vi "AlGaInPAs_prep_run_cont_dil_v14.vi"(2 "Debug Mode":bool, 3 "Elapsed Time(s)":dbl, 4 "State":enum16{"Edit", "Start", "Run", "End", "Idle"}(ring), 5 "Argument List In":string[](array[string])) -> (0 "Status Out":string, 1 "Argument List Out":string[](array[string]))   [LabVIEW 2011]
panel:
  out "Prep-In var":bool
  out "Prep-Ga var":bool
  out "Prep-Al var":bool
  out "Prep-P var":bool
  out "Prep-As var":bool
  out "prep_done":bool
  out "run started":bool
  out "first":bool=TRUE
  out "total time":dbl
  out "is OK?":bool
  out "AsH3?":bool
  out "PH3?":bool
  out "In?":bool
  out "Ga?":bool
  out "Al?":bool
  in  "Prep As":bool caption="Pre-run"
  in  "Prep P":bool caption="Pre-run"
  in  "Prep In":bool caption="Pre-run"
  in  "prep_time":dbl caption="pre-run time (s)"
  in  "Prep Al":bool caption="Pre-run"
  in  "Run As":bool caption="Run"
  in  "AsH3 Flow":dbl caption="AsH3 Flow (0-10 sccm)" format="%.2f"
  in  "P Flow":dbl caption="P Flow (0-100 sccm)" format="%.2f"
  in  "Run P":bool caption="Run"
  in  "In Flow":dbl caption="In Flow (0-100 sscm)" format="%.2f"
  in  "Run In":bool caption="Run"
  in  "Run Al":bool caption="Run"
  in  "Al Flow":dbl caption="Al Flow (0-100 sscm)" format="%.2f"
  in  "Cancel":bool
  in  "OK":bool
  out "tTotal(s) 2":dbl
  in  "Ga Tab Control":enum32{"Page 1", "Page 2", "Page 3"}(tab)
  in  "Ga Dilution":bool caption="Dilute"
  in  "Ga Flow set":dbl=1.0 caption="Ga Flow (0-10 sscm)" format="%.4f"
  in  "Run Ga":bool caption="Run"
  in  "Prep Ga":bool caption="Pre-run"
  out "Ga Flow val":dbl caption="Ga Flow (0-10 sscm)" format="%.2f"
  in  "GAMFC1 set":dbl=1.0 caption="R1 (0-10 sscm)" format="%.2f"
  in  "GAMFC3 set":dbl=100.0 caption="R3 (0-1000 sscm)" format="%.1f"
  out "GAMFC1 val":dbl caption="R1 (0-10 sscm)" format="%.2f"
  in  "GAMFC2 set":dbl=10.0 caption="R2 (0-100 sscm)" format="%.2f"
  out "GAMFC3 val":dbl=100.0 caption="R3 (0-1000 sscm)" format="%.1f"
  out "GAMFC2 val":dbl caption="R2 (0-100 sscm)" format="%.2f"
  in  "Ga calculated":u16(ring) items=["Ga flow", "MFC1", "MFC2", "MFC3"]
  # "Add pre-run time to run time in editor."
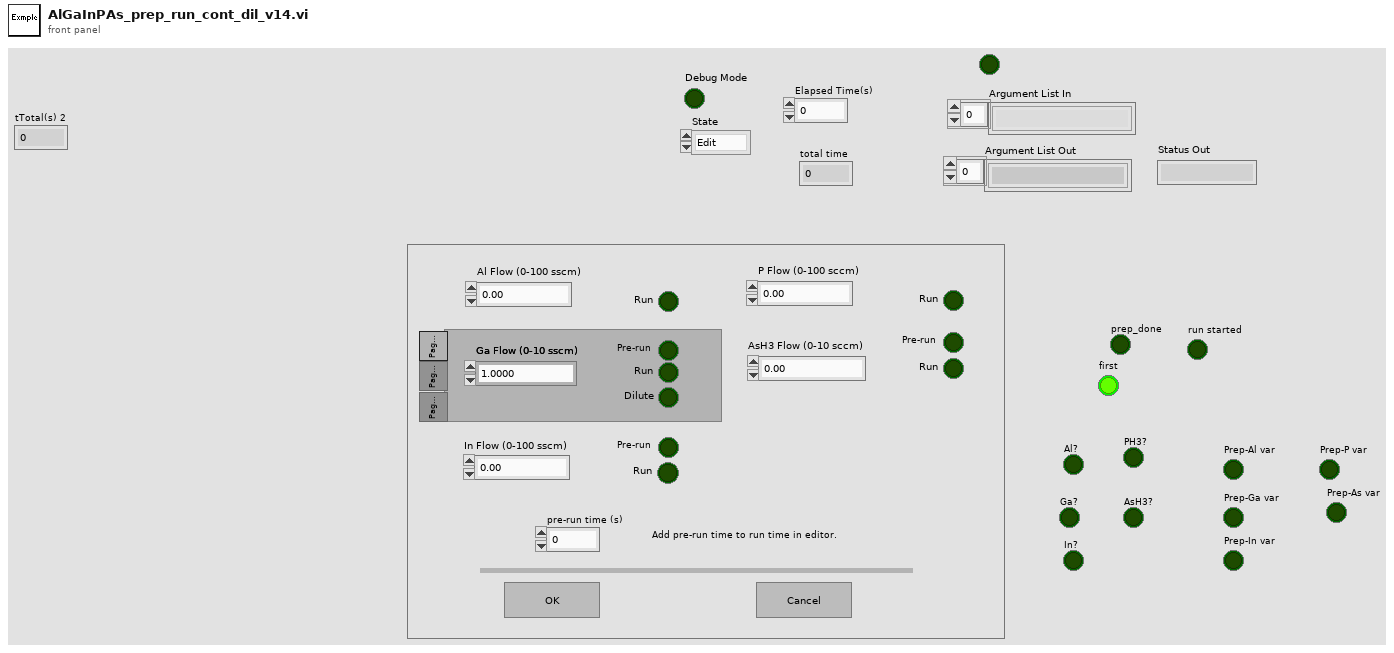
[diagram p1: front panel]
types:
  T1 = enum16{"Discrete", "Continuous", "Instantaneous", "Finite"}
  T2 = enum32{"Invalid", "Default", "Floating", "Floating/Auto-Hide", "Modal"}
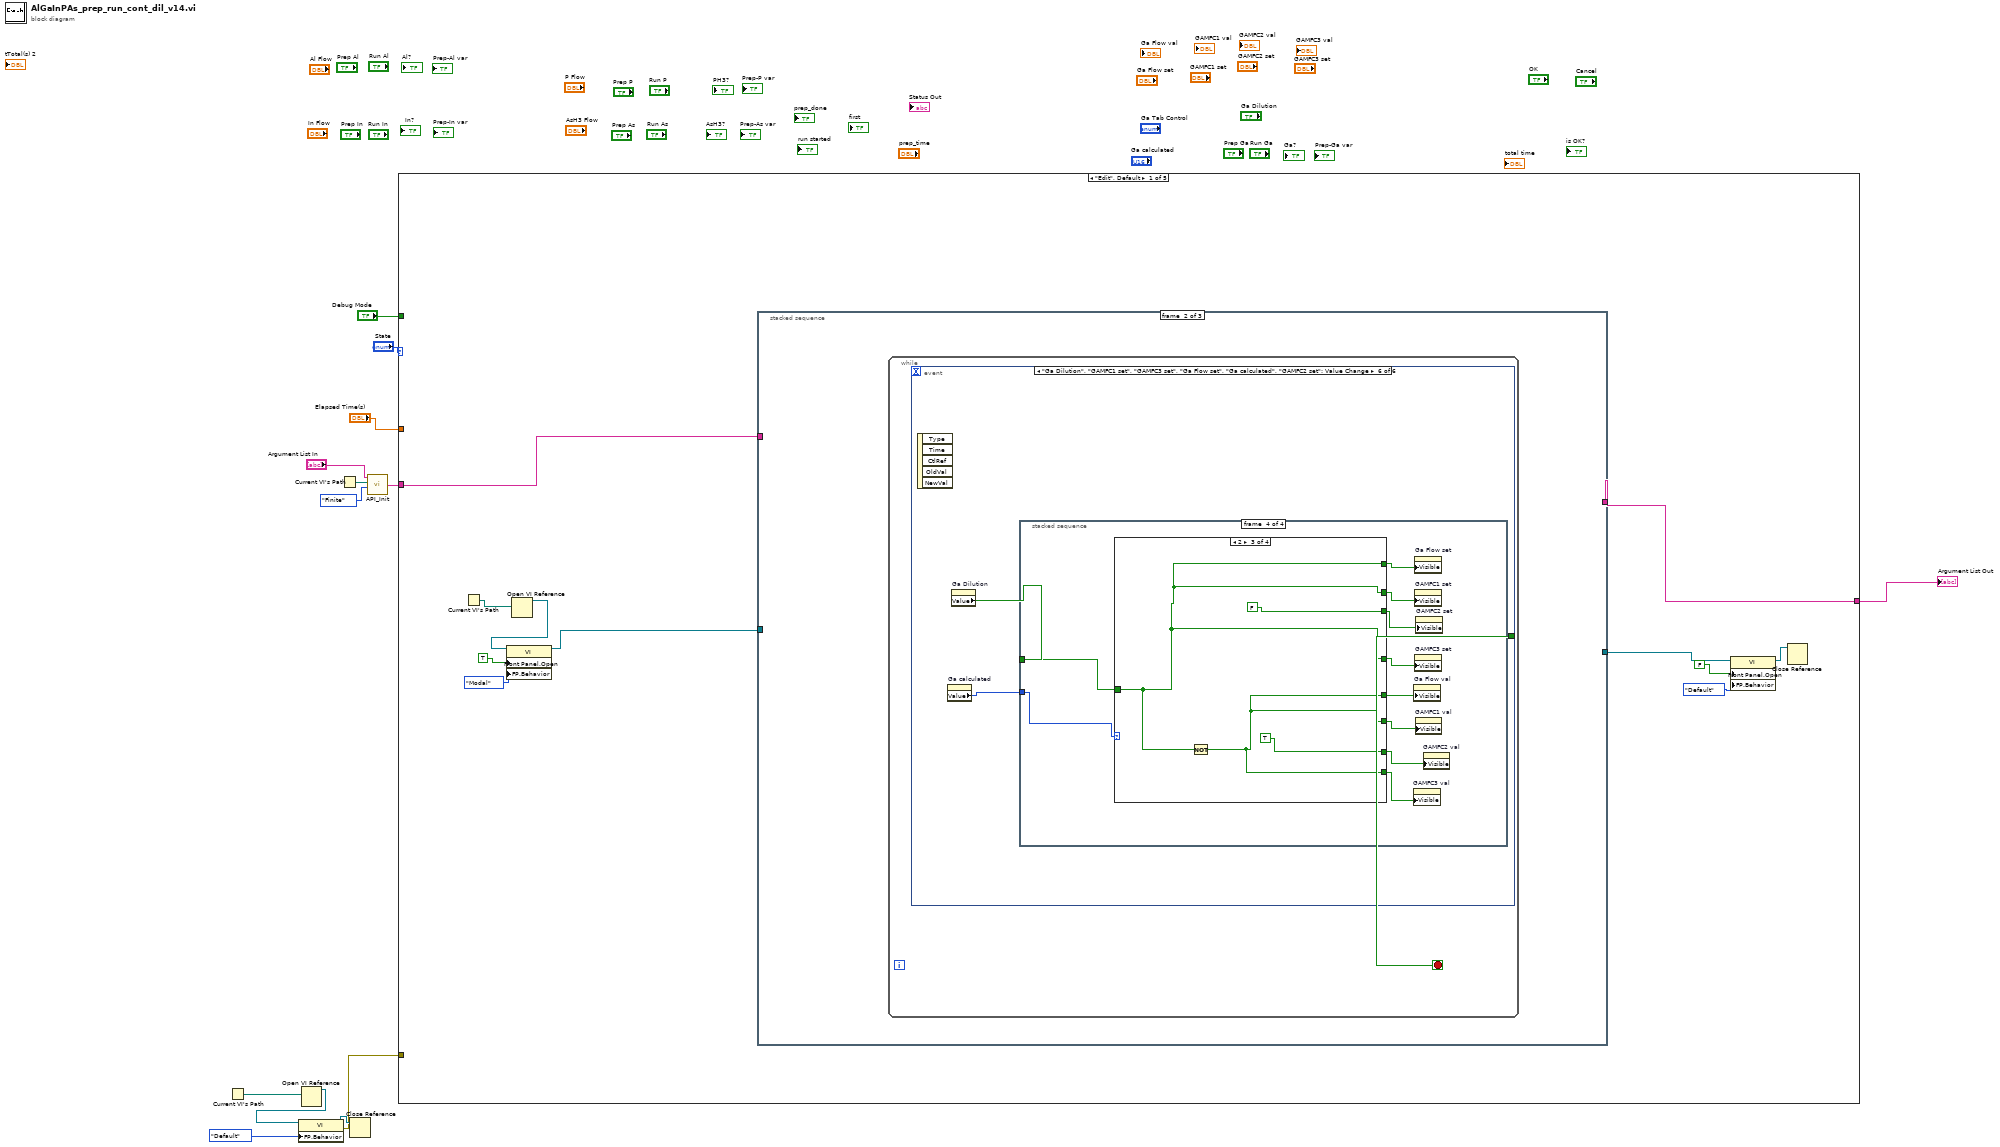
[diagram p0: block diagram]
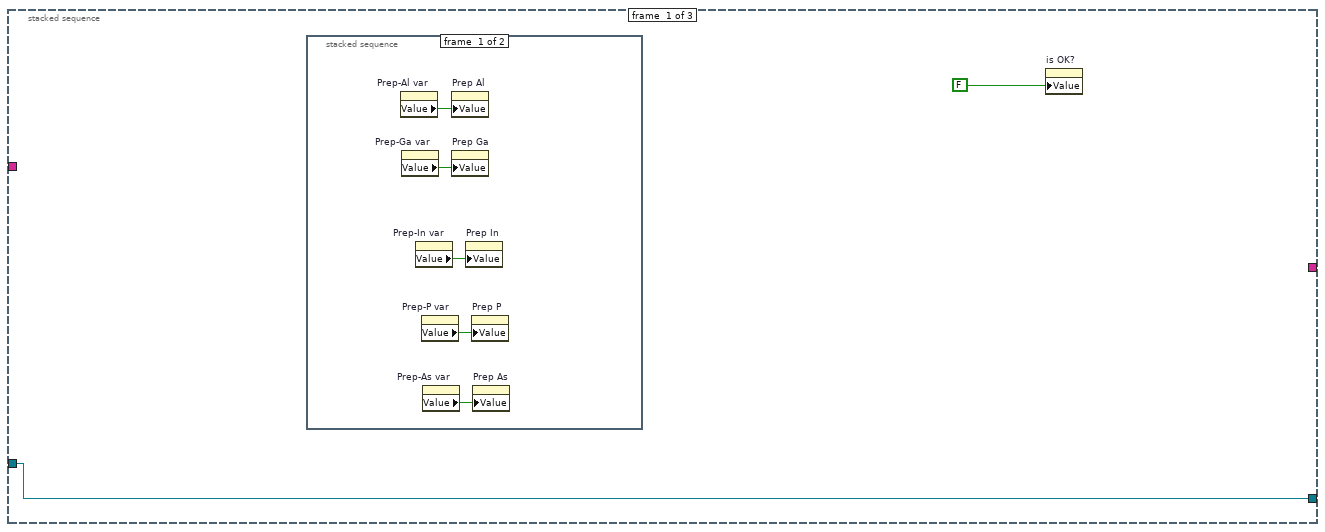
[diagram p2: hidden frame]
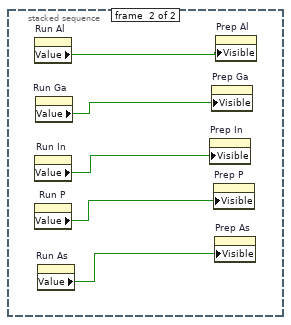
[diagram p3: hidden frame]
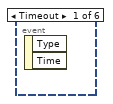
[diagram p4: hidden frame]
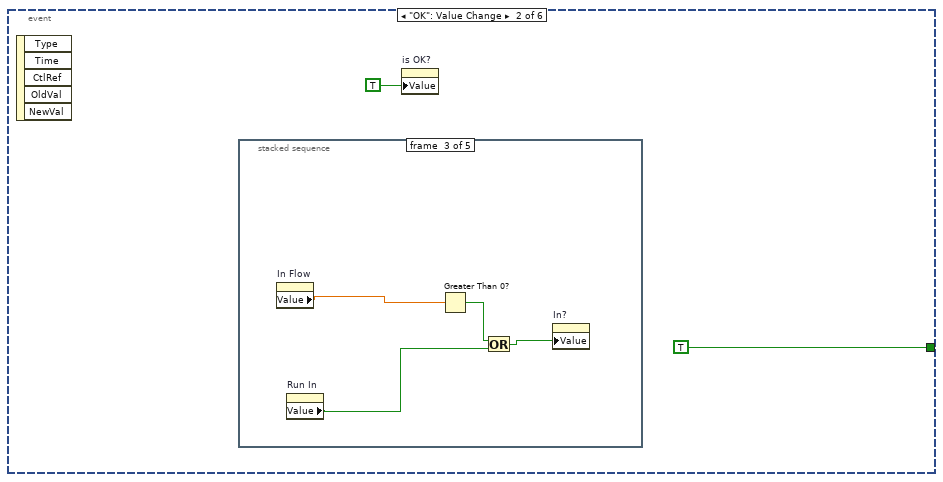
[diagram p5: hidden frame]
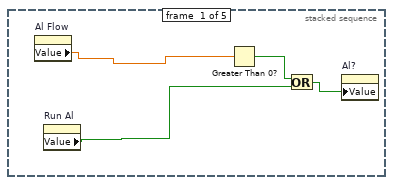
[diagram p6: hidden frame]
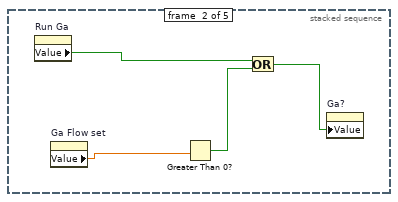
[diagram p7: hidden frame]
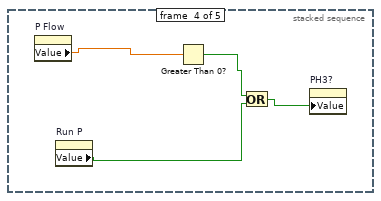
[diagram p8: hidden frame]
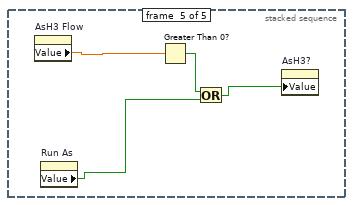
[diagram p9: hidden frame]
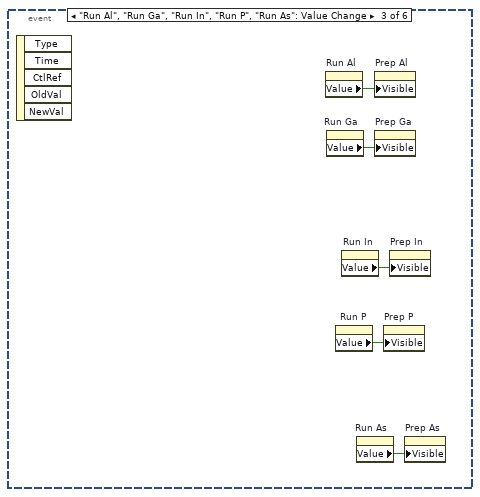
[diagram p10: hidden frame]
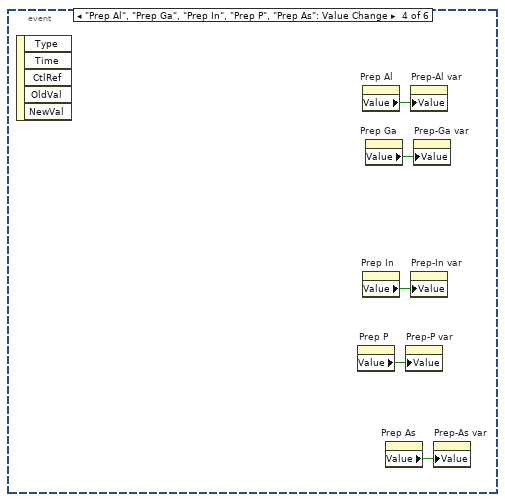
[diagram p11: hidden frame]
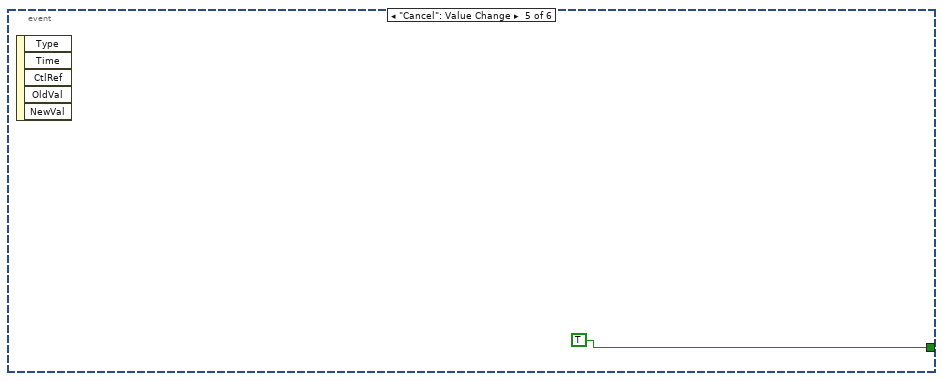
[diagram p12: hidden frame]
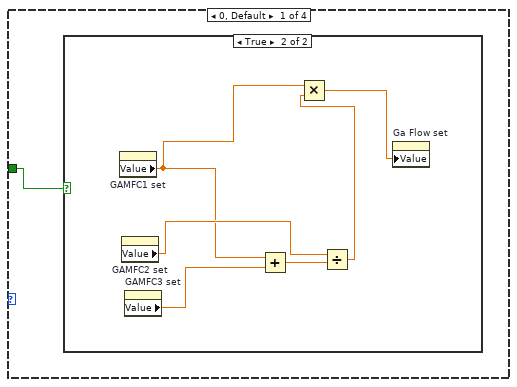
[diagram p14: hidden frame]
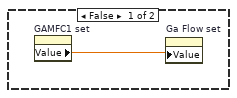
[diagram p15: hidden frame]
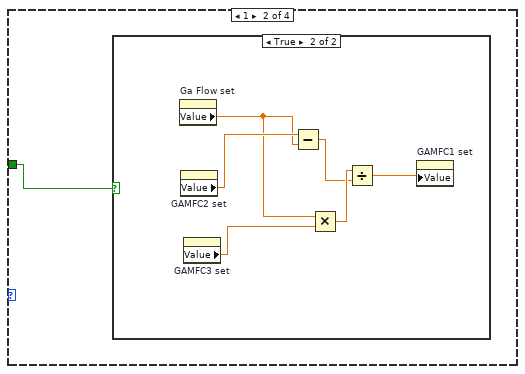
[diagram p16: hidden frame]
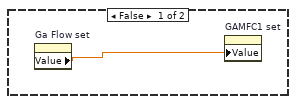
[diagram p17: hidden frame]
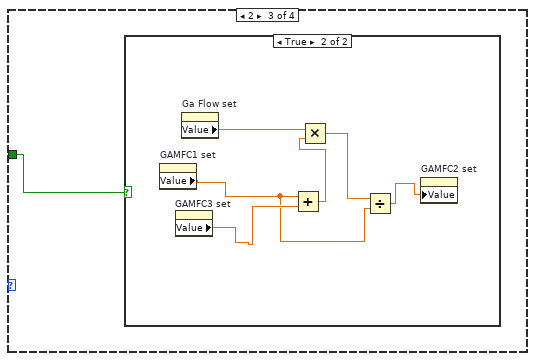
[diagram p18: hidden frame]
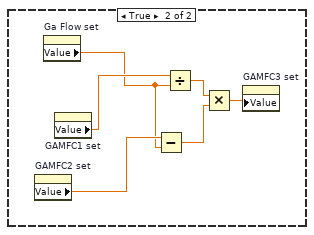
[diagram p20: hidden frame]
diagram:
  n1 = Current VI's Path() -> (path=w9:path)
  n2 = Open VI Reference(vi path=w9) -> (vi reference=w8:refnum<vi>)  [unwired: 1 in, 5 out]
  n3 = property class="VI"(reference=w8, "FP.Behavior"=T2."Default" ("Front Panel Window:Behavior")) -> (reference out=w6:refnum<vi>, error out=w5:errorcluster)  [unwired: 1 in]
  n4 = Current VI's Path() -> (path=w4:path)
  n5 = Close Reference(reference=w6) -> ()  [unwired: 1 in, 1 out]
  n6 = call "API_Init.vi"("API Mode"=T1."Finite", "VI Path"=w4, "Argument List In"="Argument List In") -> ("Argument List Out"=w1:string[])  [unwired: 1 in]
  n7 = case shown="\"Edit\", Default" "State" {
    tunnel: "Debug Mode" -> [_ w146 w200 _ _]
    tunnel: "Elapsed Time(s)" -> [_ _ w202 _ _]
    tunnel: w1 -> [w15 w148 w199 w317 w318]
    tunnel: [w14 w147 w201 w317 w318] -> w10
    tunnel: w5 -> [_ _ _ _ _]
    frame "Edit", Default {
      n8 = Current VI's Path() -> (path=w20:path)
      n9 = Open VI Reference(vi path=w20) -> (vi reference=w19:refnum<vi>)  [unwired: 1 in, 5 out]
      n10 = property class="VI"(reference=w19, "Front Panel.Open"=TRUE ("Front Panel Window:Open"), "FP.Behavior"=T2."Modal" ("Front Panel Window:Behavior")) -> (reference out=w18:refnum<vi>)  [unwired: 1 in, 1 out]
      n11 = stacked-sequence {
        tunnel: w15 -> [_ _ w141]
        tunnel: w18 -> [w26 _ _]
        tunnel: [w26 _ _] -> w22
        tunnel: [_ _ w139] -> w14
        frame #0 {
          n12 = stacked-sequence {
            frame #0 {
              n13 = property on="Prep-Al var" class="Bool (strict)"() -> ("Value"=w31:bool)  [unwired: 2 in, 2 out]
              n14 = property on="Prep-Ga var" class="Bool (strict)"() -> ("Value"=w30:bool)  [unwired: 2 in, 2 out]
              n15 = property on="Prep-In var" class="Bool (strict)"() -> ("Value"=w29:bool)  [unwired: 2 in, 2 out]
              n16 = property on="Prep-P var" class="Bool (strict)"() -> ("Value"=w28:bool)  [unwired: 2 in, 2 out]
              n17 = property on="Prep-As var" class="Bool (strict)"() -> ("Value"=w27:bool)  [unwired: 2 in, 2 out]
              n18 = property on="Prep Al" class="Bool (strict)"("Value"=w31) -> ()  [unwired: 2 in, 2 out]
              n19 = property on="Prep Ga" class="Bool (strict)"("Value"=w30) -> ()  [unwired: 2 in, 2 out]
              n20 = property on="Prep In" class="Bool (strict)"("Value"=w29) -> ()  [unwired: 2 in, 2 out]
              n21 = property on="Prep P" class="Bool (strict)"("Value"=w28) -> ()  [unwired: 2 in, 2 out]
              n22 = property on="Prep As" class="Bool (strict)"("Value"=w27) -> ()  [unwired: 2 in, 2 out]
            }
            frame #1 {
              n23 = property on="Run Al" class="Bool (strict)"() -> ("Value"=w36:bool)  [unwired: 2 in, 2 out]
              n24 = property on="Run In" class="Bool (strict)"() -> ("Value"=w34:bool)  [unwired: 2 in, 2 out]
              n25 = property on="Run P" class="Bool (strict)"() -> ("Value"=w33:bool)  [unwired: 2 in, 2 out]
              n26 = property on="Run Ga" class="Bool (strict)"() -> ("Value"=w35:bool)  [unwired: 2 in, 2 out]
              n27 = property on="Run As" class="Bool (strict)"() -> ("Value"=w32:bool)  [unwired: 2 in, 2 out]
              n28 = property on="Prep In" class="Bool (strict)"("Visible"=w34) -> ()  [unwired: 2 in, 2 out]
              n29 = property on="Prep Ga" class="Bool (strict)"("Visible"=w35) -> ()  [unwired: 2 in, 2 out]
              n30 = property on="Prep P" class="Bool (strict)"("Visible"=w33) -> ()  [unwired: 2 in, 2 out]
              n31 = property on="Prep As" class="Bool (strict)"("Visible"=w32) -> ()  [unwired: 2 in, 2 out]
              n32 = property on="Prep Al" class="Bool (strict)"("Visible"=w36) -> ()  [unwired: 2 in, 2 out]
            }
          }
          n33 = property on="is OK?" class="Bool (strict)"("Value"=FALSE ("is OK?")) -> ()  [unwired: 2 in, 2 out]
        }
        frame #1 {
          n34 = while {
            stop <- w37 stop-if-true
            n35 = event shown="[5] \"Ga Dilution\", \"GAMFC1 set\", \"GAMFC3 set\", \"Ga Flow set\", \"Ga calculated\", \"GAMFC2 set\": Value Change" {
              selector: _ -> [_ _ _ _ _ _]
              dyn-events: _ -> [_ _ _ _ _ _]
              timeout: _ -> [_ _ _ _ _ _]
              tunnel: [_ TRUE _ _ TRUE _] -> w37
              event Timeout {
                n36 = event-data() -> ()  [unwired: 1 in, 2 out]
              }
              event "OK": Value Change {
                n37 = event-data() -> ()  [unwired: 1 in, 5 out]
                n38 = stacked-sequence {
                  frame #0 {
                    n39 = property on="Al Flow" class="DigNum (strict)"() -> ("Value"=w42:dbl)  [unwired: 2 in, 2 out]
                    n40 = property on="Run Al" class="Bool (strict)"() -> ("Value"=w41:bool)  [unwired: 2 in, 2 out]
                    n41 = Greater Than 0?(x=w42) -> (x > 0?=w43:bool)
                    n42 = Or(x=w43, y=w41) -> (x .or. y?=w40:bool)
                    n43 = property on="Al?" class="Bool (strict)"("Value"=w40) -> ()  [unwired: 2 in, 2 out]
                  }
                  frame #1 {
                    n44 = property on="Run Ga" class="Bool (strict)"() -> ("Value"=w45:bool)  [unwired: 2 in, 2 out]
                    n45 = property on="Ga Flow set" class="DigNum (strict)"() -> ("Value"=w46:dbl)  [unwired: 2 in, 2 out]
                    n46 = Greater Than 0?(x=w46) -> (x > 0?=w47:bool)
                    n47 = Or(x=w45, y=w47) -> (x .or. y?=w44:bool)
                    n48 = property on="Ga?" class="Bool (strict)"("Value"=w44) -> ()  [unwired: 2 in, 2 out]
                  }
                  frame #2 {
                    n49 = property on="In Flow" class="DigNum (strict)"() -> ("Value"=w49:dbl)  [unwired: 2 in, 2 out]
                    n50 = property on="Run In" class="Bool (strict)"() -> ("Value"=w50:bool)  [unwired: 2 in, 2 out]
                    n51 = Greater Than 0?(x=w49) -> (x > 0?=w51:bool)
                    n52 = Or(x=w51, y=w50) -> (x .or. y?=w48:bool)
                    n53 = property on="In?" class="Bool (strict)"("Value"=w48) -> ()  [unwired: 2 in, 2 out]
                  }
                  frame #3 {
                    n54 = property on="P Flow" class="DigNum (strict)"() -> ("Value"=w54:dbl)  [unwired: 2 in, 2 out]
                    n55 = property on="Run P" class="Bool (strict)"() -> ("Value"=w53:bool)  [unwired: 2 in, 2 out]
                    n56 = Greater Than 0?(x=w54) -> (x > 0?=w55:bool)
                    n57 = Or(x=w55, y=w53) -> (x .or. y?=w52:bool)
                    n58 = property on="PH3?" class="Bool (strict)"("Value"=w52) -> ()  [unwired: 2 in, 2 out]
                  }
                  frame #4 {
                    n59 = property on="AsH3 Flow" class="DigNum (strict)"() -> ("Value"=w58:dbl)  [unwired: 2 in, 2 out]
                    n60 = property on="Run As" class="Bool (strict)"() -> ("Value"=w57:bool)  [unwired: 2 in, 2 out]
                    n61 = Greater Than 0?(x=w58) -> (x > 0?=w59:bool)
                    n62 = Or(x=w59, y=w57) -> (x .or. y?=w56:bool)
                    n63 = property on="AsH3?" class="Bool (strict)"("Value"=w56) -> ()  [unwired: 2 in, 2 out]
                  }
                }
                n64 = property on="is OK?" class="Bool (strict)"("Value"=TRUE ("is OK?")) -> ()  [unwired: 2 in, 2 out]
              }
              event "Run Al", "Run Ga", "Run In", "Run P", "Run As": Value Change {
                n65 = event-data() -> ()  [unwired: 1 in, 5 out]
                n66 = property on="Run Al" class="Bool (strict)"() -> ("Value"=w64:bool)  [unwired: 2 in, 2 out]
                n67 = property on="Run Ga" class="Bool (strict)"() -> ("Value"=w63:bool)  [unwired: 2 in, 2 out]
                n68 = property on="Run P" class="Bool (strict)"() -> ("Value"=w60:bool)  [unwired: 2 in, 2 out]
                n69 = property on="Run In" class="Bool (strict)"() -> ("Value"=w62:bool)  [unwired: 2 in, 2 out]
                n70 = property on="Run As" class="Bool (strict)"() -> ("Value"=w61:bool)  [unwired: 2 in, 2 out]
                n71 = property on="Prep Al" class="Bool (strict)"("Visible"=w64) -> ()  [unwired: 2 in, 2 out]
                n72 = property on="Prep Ga" class="Bool (strict)"("Visible"=w63) -> ()  [unwired: 2 in, 2 out]
                n73 = property on="Prep P" class="Bool (strict)"("Visible"=w60) -> ()  [unwired: 2 in, 2 out]
                n74 = property on="Prep In" class="Bool (strict)"("Visible"=w62) -> ()  [unwired: 2 in, 2 out]
                n75 = property on="Prep As" class="Bool (strict)"("Visible"=w61) -> ()  [unwired: 2 in, 2 out]
              }
              event "Prep Al", "Prep Ga", "Prep In", "Prep P", "Prep As": Value Change {
                n76 = event-data() -> ()  [unwired: 1 in, 5 out]
                n77 = property on="Prep P" class="Bool (strict)"() -> ("Value"=w66:bool)  [unwired: 2 in, 2 out]
                n78 = property on="Prep Al" class="Bool (strict)"() -> ("Value"=w69:bool)  [unwired: 2 in, 2 out]
                n79 = property on="Prep In" class="Bool (strict)"() -> ("Value"=w67:bool)  [unwired: 2 in, 2 out]
                n80 = property on="Prep Ga" class="Bool (strict)"() -> ("Value"=w68:bool)  [unwired: 2 in, 2 out]
                n81 = property on="Prep As" class="Bool (strict)"() -> ("Value"=w65:bool)  [unwired: 2 in, 2 out]
                n82 = property on="Prep-P var" class="Bool (strict)"("Value"=w66) -> ()  [unwired: 2 in, 2 out]
                n83 = property on="Prep-Al var" class="Bool (strict)"("Value"=w69) -> ()  [unwired: 2 in, 2 out]
                n84 = property on="Prep-In var" class="Bool (strict)"("Value"=w67) -> ()  [unwired: 2 in, 2 out]
                n85 = property on="Prep-Ga var" class="Bool (strict)"("Value"=w68) -> ()  [unwired: 2 in, 2 out]
                n86 = property on="Prep-As var" class="Bool (strict)"("Value"=w65) -> ()  [unwired: 2 in, 2 out]
              }
              event "Cancel": Value Change {
                n87 = event-data() -> ()  [unwired: 1 in, 5 out]
              }
              event "Ga Dilution", "GAMFC1 set", "GAMFC3 set", "Ga Flow set", "Ga calculated", "GAMFC2 set": Value Change {
                n88 = event-data() -> ()  [unwired: 1 in, 5 out]
                n89 = property on="Ga calculated" class="Ring (strict)"() -> ("Value"=w71:u16)  [unwired: 2 in, 2 out]
                n90 = property on="Ga Dilution" class="Bool (strict)"() -> ("Value"=w72:bool)  [unwired: 2 in, 2 out]
                n91 = stacked-sequence {
                  tunnel: w72 -> [w74 _ w109 w121]
                  tunnel: w71 -> [w73 _ _ w112]
                  frame #0 {
                    n92 = case shown="3" w73 {
                      tunnel: w74 -> [w75 w83 w91 w98]
                      frame 0, Default {
                        n93 = case shown="True" w75 {
                          frame False {
                            n94 = property on="GAMFC1 set" class="DigNum (strict)"() -> ("Value"=w76:dbl)  [unwired: 2 in, 2 out]
                            n95 = property on="Ga Flow set" class="DigNum (strict)"("Value"=w76) -> ()  [unwired: 2 in, 2 out]
                          }
                          frame True {
                            n96 = property on="GAMFC1 set" class="DigNum (strict)"() -> ("Value"=w78:dbl)  [unwired: 2 in, 2 out]
                            n97 = property on="GAMFC2 set" class="DigNum (strict)"() -> ("Value"=w80:dbl)  [unwired: 2 in, 2 out]
                            n98 = property on="GAMFC3 set" class="DigNum (strict)"() -> ("Value"=w82:dbl)  [unwired: 2 in, 2 out]
                            n99 = Add(x=w78, y=w82) -> (x+y=w81:dbl)
                            n100 = Divide(x=w80, y=w81) -> (x/y=w79:dbl)
                            n101 = Multiply(x=w78, y=w79) -> (x*y=w77:dbl)
                            n102 = property on="Ga Flow set" class="DigNum (strict)"("Value"=w77) -> ()  [unwired: 2 in, 2 out]
                          }
                        }
                      }
                      frame 1 {
                        n103 = case shown="True" w83 {
                          frame False {
                            n104 = property on="Ga Flow set" class="DigNum (strict)"() -> ("Value"=w84:dbl)  [unwired: 2 in, 2 out]
                            n105 = property on="GAMFC1 set" class="DigNum (strict)"("Value"=w84) -> ()  [unwired: 2 in, 2 out]
                          }
                          frame True {
                            n106 = property on="Ga Flow set" class="DigNum (strict)"() -> ("Value"=w89:dbl)  [unwired: 2 in, 2 out]
                            n107 = property on="GAMFC2 set" class="DigNum (strict)"() -> ("Value"=w90:dbl)  [unwired: 2 in, 2 out]
                            n108 = property on="GAMFC3 set" class="DigNum (strict)"() -> ("Value"=w88:dbl)  [unwired: 2 in, 2 out]
                            n109 = Subtract(x=w90, y=w89) -> (x-y=w86:dbl)
                            n110 = Multiply(x=w89, y=w88) -> (x*y=w87:dbl)
                            n111 = Divide(x=w87, y=w86) -> (x/y=w85:dbl)
                            n112 = property on="GAMFC1 set" class="DigNum (strict)"("Value"=w85) -> ()  [unwired: 2 in, 2 out]
                          }
                        }
                      }
                      frame 2 {
                        n113 = case shown="True" w91 {
                          frame False {
                          }
                          frame True {
                            n114 = property on="GAMFC1 set" class="DigNum (strict)"() -> ("Value"=w93:dbl)  [unwired: 2 in, 2 out]
                            n115 = property on="GAMFC3 set" class="DigNum (strict)"() -> ("Value"=w95:dbl)  [unwired: 2 in, 2 out]
                            n116 = property on="Ga Flow set" class="DigNum (strict)"() -> ("Value"=w96:dbl)  [unwired: 2 in, 2 out]
                            n117 = Add(x=w93, y=w95) -> (x+y=w97:dbl)
                            n118 = Multiply(x=w96, y=w97) -> (x*y=w94:dbl)
                            n119 = Divide(x=w94, y=w93) -> (x/y=w92:dbl)
                            n120 = property on="GAMFC2 set" class="DigNum (strict)"("Value"=w92) -> ()  [unwired: 2 in, 2 out]
                          }
                        }
                      }
                      frame 3 {
                        n121 = case shown="False" w98 {
                          frame False {
                          }
                          frame True {
                            n122 = property on="GAMFC2 set" class="DigNum (strict)"() -> ("Value"=w104:dbl)  [unwired: 2 in, 2 out]
                            n123 = property on="Ga Flow set" class="DigNum (strict)"() -> ("Value"=w102:dbl)  [unwired: 2 in, 2 out]
                            n124 = property on="GAMFC1 set" class="DigNum (strict)"() -> ("Value"=w103:dbl)  [unwired: 2 in, 2 out]
                            n125 = Subtract(x=w104, y=w102) -> (x-y=w100:dbl)
                            n126 = Divide(x=w103, y=w102) -> (x/y=w101:dbl)
                            n127 = Multiply(x=w101, y=w100) -> (x*y=w99:dbl)
                            n128 = property on="GAMFC3 set" class="DigNum (strict)"("Value"=w99) -> ()  [unwired: 2 in, 2 out]
                          }
                        }
                      }
                    }
                  }
                  frame #1 {
                    n129 = property on="GAMFC1 set" class="DigNum (strict)"() -> ("Value"=w107:dbl)  [unwired: 2 in, 2 out]
                    n130 = property on="Ga Flow set" class="DigNum (strict)"() -> ("Value"=w108:dbl)  [unwired: 2 in, 2 out]
                    n131 = property on="GAMFC2 set" class="DigNum (strict)"() -> ("Value"=w106:dbl)  [unwired: 2 in, 2 out]
                    n132 = property on="GAMFC3 set" class="DigNum (strict)"() -> ("Value"=w105:dbl)  [unwired: 2 in, 2 out]
                    n133 = property on="GAMFC3 val" class="DigNum (strict)"("Value"=w105) -> ()  [unwired: 2 in, 2 out]
                    n134 = property on="GAMFC1 val" class="DigNum (strict)"("Value"=w107) -> ()  [unwired: 2 in, 2 out]
                    n135 = property on="GAMFC2 val" class="DigNum (strict)"("Value"=w106) -> ()  [unwired: 2 in, 2 out]
                    n136 = property on="Ga Flow val" class="DigNum (strict)"("Value"=w108) -> ()  [unwired: 2 in, 2 out]
                  }
                  frame #2 {
                    n137 = case shown="True" w109 {
                      frame False {
                        n138 = property on="Ga calculated" class="Ring (strict)"("Disabled Items []"=i32[] [2, 3]) -> ()  [unwired: 2 in, 2 out]
                      }
                      frame True {
                        n139 = property on="Ga calculated" class="Ring (strict)"("Disabled Items []"=i32[] []) -> ()  [unwired: 2 in, 2 out]
                      }
                    }
                  }
                  frame #3 {
                    n140 = case shown="2" w112 {
                      tunnel: w121 -> [w124 w127 w131 w135]
                      tunnel: [FALSE ("Visible") w127 w131 w135] -> w120
                      tunnel: [w124 FALSE ("Visible") w131 w135] -> w118
                      tunnel: [w124 w127 FALSE ("Visible") w135] -> w119
                      tunnel: [w124 w127 w131 FALSE ("Visible")] -> w117
                      tunnel: [w123 TRUE ("Visible") w130 w134] -> w115
                      tunnel: [w123 w126 TRUE ("Visible") w134] -> w114
                      tunnel: [w123 w126 w130 TRUE ("Visible")] -> w113
                      tunnel: [TRUE ("Visible") w126 w130 w134] -> w116
                      frame 0, Default {
                        n141 = Not(x=w124) -> (.not. x?=w123:bool)
                      }
                      frame 1 {
                        n142 = Not(x=w127) -> (.not. x?=w126:bool)
                      }
                      frame 2 {
                        n143 = Not(x=w131) -> (.not. x?=w130:bool)
                      }
                      frame 3 {
                        n144 = Not(x=w135) -> (.not. x?=w134:bool)
                      }
                    }
                    n145 = property on="GAMFC3 val" class="DigNum (strict)"("Visible"=w113) -> ()  [unwired: 2 in, 2 out]
                    n146 = property on="Ga Flow val" class="DigNum (strict)"("Visible"=w116) -> ()  [unwired: 2 in, 2 out]
                    n147 = property on="Ga Flow set" class="DigNum (strict)"("Visible"=w120) -> ()  [unwired: 2 in, 2 out]
                    n148 = property on="GAMFC1 set" class="DigNum (strict)"("Visible"=w118) -> ()  [unwired: 2 in, 2 out]
                    n149 = property on="GAMFC3 set" class="DigNum (strict)"("Visible"=w117) -> ()  [unwired: 2 in, 2 out]
                    n150 = property on="GAMFC1 val" class="DigNum (strict)"("Visible"=w115) -> ()  [unwired: 2 in, 2 out]
                    n151 = property on="GAMFC2 set" class="DigNum (strict)"("Visible"=w119) -> ()  [unwired: 2 in, 2 out]
                    n152 = property on="GAMFC2 val" class="DigNum (strict)"("Visible"=w114) -> ()  [unwired: 2 in, 2 out]
                  }
                }
              }
            }
          }
        }
        frame #2 {
          n153 = property on="is OK?" class="Bool (strict)"() -> ("Value"=w138:bool)  [unwired: 2 in, 2 out]
          n154 = case shown="True" w138 {
            tunnel: w141 -> [w144 w145]
            tunnel: [w144 w145] -> w140
            frame False {
            }
            frame True {
            }
          }
          n155 = Not(x=w138) -> (.not. x?=w143:bool)
          n156 = Current VI's Path() -> (path=w142:path)
          n157 = call "API_Edit.vi"("Cancel"=w143, "OK"=w138, "VI Path"=w142, "Argument List In"=w140) -> ("Argument List Out"=w139:string[])
        }
      }
      n158 = property class="VI"(reference=w22, "Front Panel.Open"=FALSE ("Front Panel Window:Open"), "FP.Behavior"=T2."Default" ("Front Panel Window:Behavior")) -> (reference out=w23:refnum<vi>)  [unwired: 1 in, 1 out]
      n159 = Close Reference(reference=w23) -> ()  [unwired: 1 in, 1 out]
    }
    frame "Start" {
      n160 = call "Set_Argument.vi"("Enable"=FALSE, "Argument"="run_started", "Argument List In"=w148) -> ("Argument List Out"=w147:string[])
      n161 = stacked-sequence {
        tunnel: w146 -> [w151 w160 w172 w181 w190]
        frame #0 {
          n162 = case shown="False" w151 {
            frame False {
              n163 = property on="Al?" class="Bool (strict)"() -> ("Value"=w152:bool)  [unwired: 2 in, 2 out]
              n164 = case shown="True" w152 {
                frame False {
                  w153 = FALSE ("Al Active")
                  n165 = call "set_Al.vi"("Aluminum Flow"=0.0, "Al Remote"=w153, "Al Run"=w153, "Al Bubbler"=w153, "Al Active"=w153) -> ()  [unwired: 5 out]
                }
                frame True {
                  w159 = TRUE ("Al Active")
                  n166 = property on="Prep Al" class="Bool (strict)"() -> ("Value"=w157:bool)  [unwired: 2 in, 2 out]
                  n167 = property on="Run Al" class="Bool (strict)"() -> ("Value"=w156:bool)  [unwired: 2 in, 2 out]
                  n168 = property on="Al Flow" class="DigNum (strict)"() -> ("Value"=w158:dbl)  [unwired: 2 in, 2 out]
                  n169 = And(x=w157, y=w156) -> (x .and. y?=w155:bool)
                  n170 = call "set_Al.vi"("Aluminum Flow"=w158, "Al Run"=w155, "Al Bubbler"=w159, "Al Active"=w159) -> ()  [unwired: 1 in, 5 out]
                }
              }
            }
            frame True {
            }
          }
        }
        frame #1 {
          n171 = case shown="False" w160 {
            frame False {
              n172 = property on="Ga?" class="Bool (strict)"() -> ("Value"=w161:bool)  [unwired: 2 in, 2 out]
              n173 = case shown="True" w161 {
                frame False {
                  w163 = FALSE ("Ga Active")
                  w162 = 0.0 ("Ga Flow 1")
                  n174 = call "set_Ga.vi"("Ga Active"=w163, "Ga Flow 3"=w162, "Ga Flow 2"=w162, "Ga Flow 1"=w162, "Ga Bubbler"=w163, "Ga H2 Dilute"=w163, "Ga Run"=w163, "Ga Remote"=w163) -> ()  [unwired: 8 out]
                }
                frame True {
                  w166 = TRUE ("Ga Active")
                  n175 = property on="GAMFC3 val" class="DigNum (strict)"() -> ("Value"=w165:dbl)  [unwired: 2 in, 2 out]
                  n176 = property on="GAMFC2 val" class="DigNum (strict)"() -> ("Value"=w167:dbl)  [unwired: 2 in, 2 out]
                  n177 = property on="Prep-Ga var" class="Bool (strict)"() -> ("Value"=w168:bool)  [unwired: 2 in, 2 out]
                  n178 = property on="GAMFC1 val" class="DigNum (strict)"() -> ("Value"=w164:dbl)  [unwired: 2 in, 2 out]
                  n179 = property on="Run Ga" class="Bool (strict)"() -> ("Value"=w169:bool)  [unwired: 2 in, 2 out]
                  n180 = And(x=w168, y=w169) -> (x .and. y?=w171:bool)
                  n181 = property on="Ga Dilution" class="Bool (strict)"() -> ("Value"=w170:bool)  [unwired: 2 in, 2 out]
                  n182 = call "set_Ga.vi"("Ga Active"=w166, "Ga Flow 3"=w165, "Ga Flow 2"=w167, "Ga Flow 1"=w164, "Ga Bubbler"=w166, "Ga H2 Dilute"=w170, "Ga Run"=w171, "Ga Remote"=w166) -> ()  [unwired: 8 in]
                }
              }
            }
            frame True {
            }
          }
        }
        frame #2 {
          n183 = case shown="False" w172 {
            frame False {
              n184 = property on="In?" class="Bool (strict)"() -> ("Value"=w173:bool)  [unwired: 2 in, 2 out]
              n185 = case shown="True" w173 {
                frame False {
                  w175 = FALSE ("In Remote")
                  n186 = call "set_In.vi"("Indium Flow"=0.0, "In Remote"=w175, "In Run"=w175, "In Bubbler"=w175, "In Active"=w175) -> ()  [unwired: 5 out]
                }
                frame True {
                  w180 = TRUE ("In Run")
                  n187 = property on="Run In" class="Bool (strict)"() -> ("Value"=w177:bool)  [unwired: 2 in, 2 out]
                  n188 = property on="Prep In" class="Bool (strict)"() -> ("Value"=w178:bool)  [unwired: 2 in, 2 out]
                  n189 = And(x=w178, y=w177) -> (x .and. y?=w176:bool)
                  n190 = property on="In Flow" class="DigNum (strict)"() -> ("Value"=w179:dbl)  [unwired: 2 in, 2 out]
                  n191 = call "set_In.vi"("Indium Flow"=w179, "In Run"=w176, "In Bubbler"=w180, "In Active"=w180) -> ()  [unwired: 1 in, 5 out]
                }
              }
            }
            frame True {
            }
          }
        }
        frame #3 {
          n192 = case shown="False" w181 {
            frame False {
              n193 = property on="PH3?" class="Bool (strict)"() -> ("Value"=w182:bool)  [unwired: 2 in, 2 out]
              n194 = case shown="True" w182 {
                frame False {
                  w183 = FALSE ("P_Gas Active")
                  n195 = call "set_P_gas.vi"("P_Gas Active"=w183, "P_Gas Flow"=0.0, "P_Gas In"=w183, "P_Gas H2 In"=w183, "P_Gas Run"=w183, "P_Gas Remote"=w183) -> ()  [unwired: 10 out]
                }
                frame True {
                  w189 = TRUE ("P_Gas Active")
                  n196 = property on="P Flow" class="DigNum (strict)"() -> ("Value"=w188:dbl)  [unwired: 2 in, 2 out]
                  n197 = property on="Prep P" class="Bool (strict)"() -> ("Value"=w187:bool)  [unwired: 2 in, 2 out]
                  n198 = property on="Run P" class="Bool (strict)"() -> ("Value"=w186:bool)  [unwired: 2 in, 2 out]
                  n199 = And(x=w187, y=w186) -> (x .and. y?=w185:bool)
                  n200 = call "set_P_gas.vi"("P_Gas Active"=w189, "P_Gas Flow"=w188, "P_Gas In"=w189, "P_Gas Run"=w185) -> ()  [unwired: 2 in, 10 out]
                }
              }
            }
            frame True {
            }
          }
        }
        frame #4 {
          n201 = case shown="False" w190 {
            frame False {
              n202 = property on="AsH3?" class="Bool (strict)"() -> ("Value"=w191:bool)  [unwired: 2 in, 2 out]
              n203 = case shown="True" w191 {
                frame False {
                  w192 = FALSE ("As_Gas Active")
                  n204 = call "set_As_gas.vi"("As_Gas Active"=w192, "As_Gas Flow"=0.0, "As_Gas In"=w192, "As_Gas H2"=w192, "As_Gas Run"=w192, "As_Gas Remote"=w192) -> ()  [unwired: 10 in]
                }
                frame True {
                  w198 = TRUE ("As_Gas Active")
                  n205 = property on="Prep As" class="Bool (strict)"() -> ("Value"=w195:bool)  [unwired: 2 in, 2 out]
                  n206 = property on="Run As" class="Bool (strict)"() -> ("Value"=w196:bool)  [unwired: 2 in, 2 out]
                  n207 = property on="AsH3 Flow" class="DigNum (strict)"() -> ("Value"=w197:dbl)  [unwired: 2 in, 2 out]
                  n208 = And(x=w195, y=w196) -> (x .and. y?=w194:bool)
                  n209 = call "set_As_gas.vi"("As_Gas Active"=w198, "As_Gas Flow"=w197, "As_Gas In"=w198, "As_Gas Run"=w194) -> ()  [unwired: 12 in]
                }
              }
            }
            frame True {
            }
          }
        }
      }
    }
    frame "Run" {
      n210 = stacked-sequence {
        tunnel: w202 -> [_ w207 _ _]
        tunnel: w199 -> [w204 _ _ w261]
        tunnel: [_ _ _ w260] -> w201
        tunnel: w200 -> [_ _ _ w262]
        frame #0 {
          n211 = call "Get_Argument.vi"("Argument"="run_started", "Argument List"=w204) -> ("Enabled"=w203:bool)
          n212 = local write "run started"(w203) -> ()
        }
        frame #1 {
          n213 = property on="prep_time" class="DigNum (strict)"() -> ("Value"=w208:dbl)  [unwired: 2 in, 2 out]
          n214 = Greater Or Equal?(x=w207, y=w208) -> (x >= y?=w206:bool)
          n215 = local write "prep_done"(w206) -> ()
        }
        frame #2 {
          n216 = local read "run started"() -> (w210:bool)
          n217 = Not(x=w210) -> (.not. x?=w209:bool)
          n218 = stacked-sequence {
            tunnel: w209 -> [w212 w216 w225 w234 w243 w252]
            frame #0 {
              n219 = case shown="True" w212 {
                tunnel: ["run: " "pre-run: "] -> w211
                frame False {
                }
                frame True {
                }
              }
              n220 = property on="Status Out" class="Str"("Value"=w211) -> ()  [unwired: 2 in, 2 out]
            }
            frame #1 {
              n221 = property on="Status Out" class="Str"() -> ("Value"=w222:string)  [unwired: 2 in, 2 out]
              n222 = property on="Al?" class="Bool (strict)"() -> ("Value"=w223:bool)  [unwired: 2 in, 2 out]
              n223 = property on="Run Al" class="Bool (strict)"() -> ("Value"=w215:bool)  [unwired: 2 in, 2 out]
              n224 = property on="Prep Al" class="Bool (strict)"() -> ("Value"=w217:bool)  [unwired: 2 in, 2 out]
              n225 = call "flow_strings.vi"("string in"=w222, "is first in?"=TRUE, "use source?"=w223, "name"="Al", "run source?"=w215, "prep source?"=w217, "is prep?"=w216) -> ("string out"=w221:string, "is first out?"=w220:bool)
              n226 = property on="Status Out" class="Str"("Value"=w221) -> ()  [unwired: 2 in, 2 out]
              n227 = property on="first" class="Bool (strict)"("Value"=w220) -> ()  [unwired: 2 in, 2 out]
            }
            frame #2 {
              n228 = property on="first" class="Bool (strict)"() -> ("Value"=w228:bool)  [unwired: 2 in, 2 out]
              n229 = property on="Status Out" class="Str"() -> ("Value"=w231:string)  [unwired: 2 in, 2 out]
              n230 = property on="Ga?" class="Bool (strict)"() -> ("Value"=w229:bool)  [unwired: 2 in, 2 out]
              n231 = property on="Run Ga" class="Bool (strict)"() -> ("Value"=w224:bool)  [unwired: 2 in, 2 out]
              n232 = property on="Prep Ga" class="Bool (strict)"() -> ("Value"=w226:bool)  [unwired: 2 in, 2 out]
              n233 = call "flow_strings.vi"("string in"=w231, "is first in?"=w228, "use source?"=w229, "name"="Ga", "run source?"=w224, "prep source?"=w226, "is prep?"=w225) -> ("string out"=w232:string, "is first out?"=w227:bool)
              n234 = property on="Status Out" class="Str"("Value"=w232) -> ()  [unwired: 2 in, 2 out]
              n235 = property on="first" class="Bool (strict)"("Value"=w227) -> ()  [unwired: 2 in, 2 out]
            }
            frame #3 {
              n236 = property on="first" class="Bool (strict)"() -> ("Value"=w238:bool)  [unwired: 2 in, 2 out]
              n237 = property on="Status Out" class="Str"() -> ("Value"=w240:string)  [unwired: 2 in, 2 out]
              n238 = property on="In?" class="Bool (strict)"() -> ("Value"=w241:bool)  [unwired: 2 in, 2 out]
              n239 = property on="Run In" class="Bool (strict)"() -> ("Value"=w233:bool)  [unwired: 2 in, 2 out]
              n240 = property on="Prep In" class="Bool (strict)"() -> ("Value"=w235:bool)  [unwired: 2 in, 2 out]
              n241 = call "flow_strings.vi"("string in"=w240, "is first in?"=w238, "use source?"=w241, "name"="In", "run source?"=w233, "prep source?"=w235, "is prep?"=w234) -> ("string out"=w237:string, "is first out?"=w236:bool)
              n242 = property on="Status Out" class="Str"("Value"=w237) -> ()  [unwired: 2 in, 2 out]
              n243 = property on="first" class="Bool (strict)"("Value"=w236) -> ()  [unwired: 2 in, 2 out]
            }
            frame #4 {
              n244 = property on="first" class="Bool (strict)"() -> ("Value"=w246:bool)  [unwired: 2 in, 2 out]
              n245 = property on="Status Out" class="Str"() -> ("Value"=w248:string)  [unwired: 2 in, 2 out]
              n246 = property on="PH3?" class="Bool (strict)"() -> ("Value"=w249:bool)  [unwired: 2 in, 2 out]
              n247 = property on="Run P" class="Bool (strict)"() -> ("Value"=w242:bool)  [unwired: 2 in, 2 out]
              n248 = property on="Prep P" class="Bool (strict)"() -> ("Value"=w244:bool)  [unwired: 2 in, 2 out]
              n249 = call "flow_strings.vi"("string in"=w248, "is first in?"=w246, "use source?"=w249, "name"="P", "run source?"=w242, "prep source?"=w244, "is prep?"=w243) -> ("string out"=w247:string, "is first out?"=w245:bool)
              n250 = property on="Status Out" class="Str"("Value"=w247) -> ()  [unwired: 2 in, 2 out]
              n251 = property on="first" class="Bool (strict)"("Value"=w245) -> ()  [unwired: 2 in, 2 out]
            }
            frame #5 {
              n252 = property on="first" class="Bool (strict)"() -> ("Value"=w255:bool)  [unwired: 2 in, 2 out]
              n253 = property on="Status Out" class="Str"() -> ("Value"=w257:string)  [unwired: 2 in, 2 out]
              n254 = property on="AsH3?" class="Bool (strict)"() -> ("Value"=w258:bool)  [unwired: 2 in, 2 out]
              n255 = property on="Run As" class="Bool (strict)"() -> ("Value"=w251:bool)  [unwired: 2 in, 2 out]
              n256 = property on="Prep As" class="Bool (strict)"() -> ("Value"=w253:bool)  [unwired: 2 in, 2 out]
              n257 = call "flow_strings.vi"("string in"=w257, "is first in?"=w255, "use source?"=w258, "name"="As", "run source?"=w251, "prep source?"=w253, "is prep?"=w252) -> ("string out"=w254:string, "is first out?"=w256:bool)
              n258 = property on="Status Out" class="Str"("Value"=w254) -> ()  [unwired: 2 in, 2 out]
              n259 = property on="first" class="Bool (strict)"("Value"=w256) -> ()  [unwired: 2 in, 2 out]
            }
          }
        }
        frame #3 {
          n260 = local read "run started"() -> (w265:bool)
          n261 = local read "prep_done"() -> (w263:bool)
          n262 = Not(x=w265) -> (.not. x?=w266:bool)
          n263 = And(x=w263, y=w266) -> (x .and. y?=w264:bool)
          n264 = stacked-sequence {
            tunnel: w264 -> [w270]
            tunnel: w262 -> [w269]
            tunnel: w261 -> [w268]
            tunnel: [w267] -> w260
            frame #0 {
              n265 = case shown="True" w270 {
                tunnel: w269 -> [_ w274]
                tunnel: w268 -> [w271 w273]
                tunnel: [w271 w272] -> w267
                frame False {
                }
                frame True {
                  n266 = stacked-sequence {
                    tunnel: w274 -> [w275 w282 w292 w299 w306 _]
                    tunnel: w273 -> [_ _ _ _ _ w314]
                    tunnel: [_ _ _ _ _ w313] -> w272
                    frame #0 {
                      n267 = case shown="False" w275 {
                        frame False {
                          n268 = property on="Al?" class="Bool (strict)"() -> ("Value"=w276:bool)  [unwired: 2 in, 2 out]
                          n269 = case shown="True" w276 {
                            frame False {
                              w277 = FALSE ("Al Active")
                              n270 = call "set_Al.vi"("Aluminum Flow"=0.0, "Al Remote"=w277, "Al Run"=w277, "Al Bubbler"=w277, "Al Active"=w277) -> ()  [unwired: 5 out]
                            }
                            frame True {
                              w281 = TRUE ("Al Active")
                              n271 = property on="Al Flow" class="DigNum (strict)"() -> ("Value"=w280:dbl)  [unwired: 2 in, 2 out]
                              n272 = property on="Run Al" class="Bool (strict)"() -> ("Value"=w279:bool)  [unwired: 2 in, 2 out]
                              n273 = call "set_Al.vi"("Aluminum Flow"=w280, "Al Run"=w279, "Al Bubbler"=w281, "Al Active"=w281) -> ()  [unwired: 1 in, 5 out]
                            }
                          }
                        }
                        frame True {
                        }
                      }
                    }
                    frame #1 {
                      n274 = case shown="False" w282 {
                        frame False {
                          n275 = property on="Ga?" class="Bool (strict)"() -> ("Value"=w283:bool)  [unwired: 2 in, 2 out]
                          n276 = case shown="True" w283 {
                            frame False {
                              w285 = FALSE ("Ga Active")
                              w284 = 0.0 ("Ga Flow 1")
                              n277 = call "set_Ga.vi"("Ga Active"=w285, "Ga Flow 3"=w284, "Ga Flow 2"=w284, "Ga Flow 1"=w284, "Ga Bubbler"=w285, "Ga H2 Dilute"=w285, "Ga Run"=w285, "Ga Remote"=w285) -> ()  [unwired: 8 out]
                            }
                            frame True {
                              w289 = TRUE ("Ga Active")
                              n278 = property on="Ga Dilution" class="Bool (strict)"() -> ("Value"=w288:bool)  [unwired: 2 in, 2 out]
                              n279 = property on="GAMFC3 val" class="DigNum (strict)"() -> ("Value"=w287:dbl)  [unwired: 2 in, 2 out]
                              n280 = property on="Run Ga" class="Bool (strict)"() -> ("Value"=w290:bool)  [unwired: 2 in, 2 out]
                              n281 = property on="GAMFC2 val" class="DigNum (strict)"() -> ("Value"=w291:dbl)  [unwired: 2 in, 2 out]
                              n282 = property on="GAMFC1 val" class="DigNum (strict)"() -> ("Value"=w286:dbl)  [unwired: 2 in, 2 out]
                              n283 = call "set_Ga.vi"("Ga Active"=w289, "Ga Flow 3"=w287, "Ga Flow 2"=w291, "Ga Flow 1"=w286, "Ga Bubbler"=w289, "Ga H2 Dilute"=w288, "Ga Run"=w290, "Ga Remote"=w289) -> ()  [unwired: 8 in]
                            }
                          }
                        }
                        frame True {
                        }
                      }
                    }
                    frame #2 {
                      n284 = case shown="False" w292 {
                        frame False {
                          n285 = property on="In?" class="Bool (strict)"() -> ("Value"=w293:bool)  [unwired: 2 in, 2 out]
                          n286 = case shown="True" w293 {
                            frame False {
                              w295 = FALSE ("In Remote")
                              n287 = call "set_In.vi"("Indium Flow"=0.0, "In Remote"=w295, "In Run"=w295, "In Bubbler"=w295, "In Active"=w295) -> ()  [unwired: 5 out]
                            }
                            frame True {
                              w298 = TRUE ("In Run")
                              n288 = property on="Run In" class="Bool (strict)"() -> ("Value"=w296:bool)  [unwired: 2 in, 2 out]
                              n289 = property on="In Flow" class="DigNum (strict)"() -> ("Value"=w297:dbl)  [unwired: 2 in, 2 out]
                              n290 = call "set_In.vi"("Indium Flow"=w297, "In Run"=w296, "In Bubbler"=w298, "In Active"=w298) -> ()  [unwired: 1 in, 5 out]
                            }
                          }
                        }
                        frame True {
                        }
                      }
                    }
                    frame #3 {
                      n291 = case shown="False" w299 {
                        frame False {
                          n292 = property on="PH3?" class="Bool (strict)"() -> ("Value"=w300:bool)  [unwired: 2 in, 2 out]
                          n293 = case shown="False" w300 {
                            frame False {
                              w301 = FALSE ("P_Gas Active")
                              n294 = call "set_P_gas.vi"("P_Gas Active"=w301, "P_Gas Flow"=0.0, "P_Gas In"=w301, "P_Gas H2 In"=w301, "P_Gas Run"=w301, "P_Gas Remote"=w301) -> ()  [unwired: 10 out]
                            }
                            frame True {
                              w305 = TRUE ("P_Gas Active")
                              n295 = property on="P Flow" class="DigNum (strict)"() -> ("Value"=w304:dbl)  [unwired: 2 in, 2 out]
                              n296 = property on="Run P" class="Bool (strict)"() -> ("Value"=w303:bool)  [unwired: 2 in, 2 out]
                              n297 = call "set_P_gas.vi"("P_Gas Active"=w305, "P_Gas Flow"=w304, "P_Gas In"=w305, "P_Gas Run"=w303) -> ()  [unwired: 2 in, 10 out]
                            }
                          }
                        }
                        frame True {
                        }
                      }
                    }
                    frame #4 {
                      n298 = case shown="False" w306 {
                        frame False {
                          n299 = property on="AsH3?" class="Bool (strict)"() -> ("Value"=w307:bool)  [unwired: 2 in, 2 out]
                          n300 = case shown="True" w307 {
                            frame False {
                              w308 = FALSE ("As_Gas Active")
                              n301 = call "set_As_gas.vi"("As_Gas Active"=w308, "As_Gas Flow"=0.0, "As_Gas In"=w308, "As_Gas H2"=w308, "As_Gas Run"=w308, "As_Gas Remote"=w308) -> ()  [unwired: 10 in]
                            }
                            frame True {
                              w311 = TRUE ("As_Gas Active")
                              n302 = property on="Run As" class="Bool (strict)"() -> ("Value"=w310:bool)  [unwired: 2 in, 2 out]
                              n303 = property on="AsH3 Flow" class="DigNum (strict)"() -> ("Value"=w312:dbl)  [unwired: 2 in, 2 out]
                              n304 = call "set_As_gas.vi"("As_Gas Active"=w311, "As_Gas Flow"=w312, "As_Gas In"=w311, "As_Gas Run"=w310) -> ()  [unwired: 12 in]
                            }
                          }
                        }
                        frame True {
                        }
                      }
                    }
                    frame #5 {
                      n305 = call "Set_Argument.vi"("Enable"=TRUE, "Argument"="run_started", "Argument List In"=w314) -> ("Argument List Out"=w313:string[])
                    }
                  }
                }
              }
            }
          }
        }
      }
    }
    frame "End" {
    }
    frame "Idle" {
    }
  }
  "Argument List Out" <- w10
